vi "BP - Assign DIO bits for jog mode.vi"(2 "Set DIO bit # (first #) to jog\naxis # above in the negative\ndirection and DIO bit # \n(,second #) to jog axis #\nabove in the positive direction":string, 3 "error in":errorcluster, 4 "Action":bool, 5 "Axis":i8=1 min=1 max=6 step=1, 6 "Address / Port":i16=1 min=1 max=31 step=1) -> (0 "error out":errorcluster, 1 "Report the DIO\nbits assigned\nfor jogging":string)   [LabVIEW 2014]
panel:
  # "Read"
  # "Write"
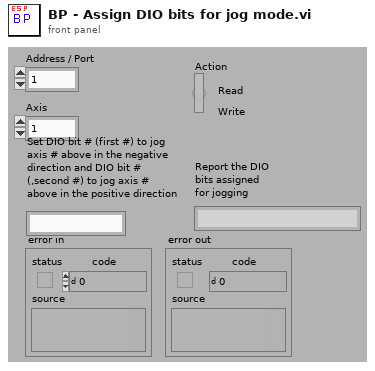
[diagram p1: front panel]
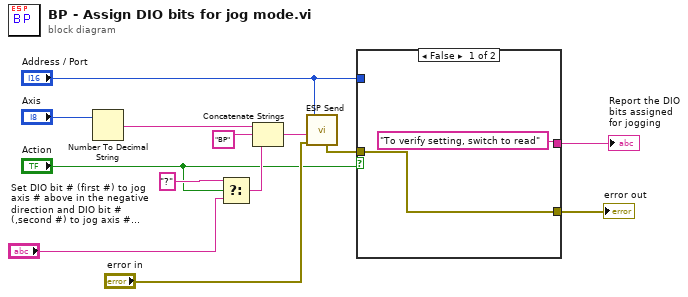
[diagram p0: block diagram]
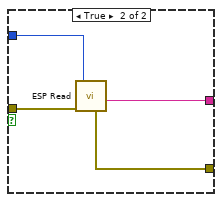
[diagram p2: hidden frame]
diagram:
  n1 = Number To Decimal String(number="Axis") -> (decimal integer string=w12:string)  [unwired: 1 in]
  n2 = Select(t="?", s="Action", f="Set DIO bit # (first #) to jog\naxis # above in the negative\ndirection and DIO bit # \n(,second #) to jog axis #\nabove in the positive direction") -> (s? t:f=w9:string)
  n3 = Concatenate Strings(w12, "BP" ("Substring"), w9) -> (w10:string)
  n4 = call "ESP Send.vi"("Address / Port"="Address / Port", "Command String"=w10, "error in"="error in") -> ("error out"=w4:errorcluster)  [unwired: 5 in]
  n5 = case shown="False" "Action" {
    tunnel: "Address / Port" -> [_ w19]
    tunnel: w4 -> [w15 w18]
    tunnel: [w15 w17] -> w3
    tunnel: ["To verify setting, switch to read" w16] -> w1
    frame False {
    }
    frame True {
      n6 = call "ESP Read.vi"("Address / Port"=w19, "error in"=w18) -> ("error out"=w17:errorcluster, "Response String"=w16:string)  [unwired: 5 in]
    }
  }
  "error out" <- w3
  "Report the DIO\nbits assigned\nfor jogging" <- w1
